vi "sCombine Slow.vi"(1 "HV Cluster":T2={"HV Power On/Off"=[], "Set Voltage"=[], "HV Tolerance (%)"=1.0}, 2 "Rad7 On?":bool, 3 "Slow Cluster":T1) -> (0 "Slow Cluster 2":T1)   [LabVIEW 2012]
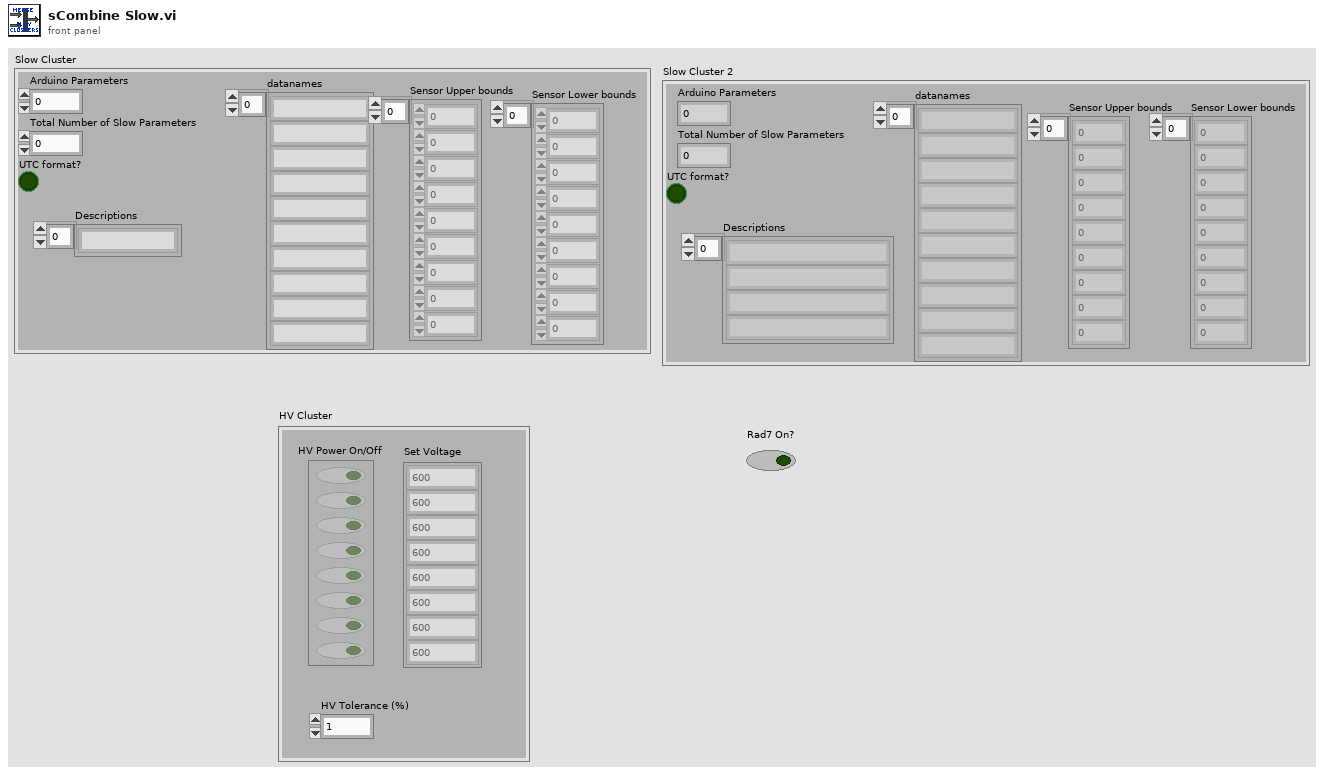
[diagram p1: front panel]
types:
  T1 = cluster{"Arduino Parameters":dbl, "Total Number of Slow Parameters":i32, "UTC format?":bool, "Sensor Upper bounds":i32[], "Sensor Lower bounds":i32[], "Descriptions":string[], "datanames":string[]}
  T2 = cluster{"HV Power On/Off":bool[], "Set Voltage":string[], "HV Tolerance (%)":dbl}
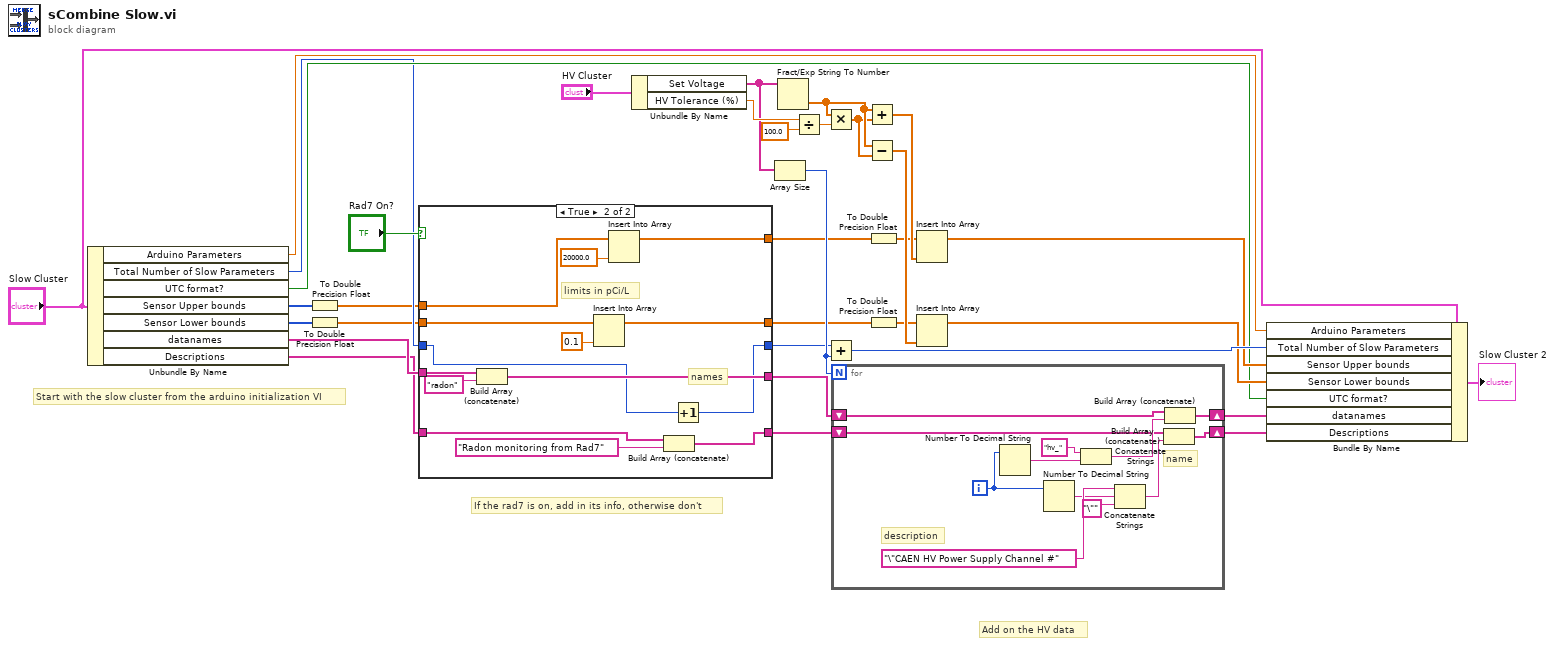
[diagram p0: block diagram]
diagram:
  # "Add on the HV data"
  # "If the rad7 is on, add in its info, otherwise don't"
  # "Start with the slow cluster from the arduino initialization VI"
  n1 = Unbundle By Name("Slow Cluster") -> ("Arduino Parameters"=w16:dbl, "Total Number of Slow Parameters"=w8:i32, "UTC format?"=w20:bool, "Sensor Upper bounds"=w4:i32[], "Sensor Lower bounds"=w3:i32[], "datanames"=w12:string[], "Descriptions"=w10:string[])
  n2 = To Double Precision Float(number=w4) -> (double precision float=w2:dbl[])
  n3 = To Double Precision Float(number=w3) -> (double precision float=w1:dbl[])
  n4 = case shown="True" "Rad7 On?" {
    tunnel: w12 -> [w39 w53]
    tunnel: [w39 w51] -> w11
    tunnel: w10 -> [w38 w49]
    tunnel: [w38 w48] -> w9
    tunnel: w8 -> [w37 w47]
    tunnel: [w37 w46] -> w7
    tunnel: w2 -> [w36 w45]
    tunnel: w1 -> [w35 w44]
    tunnel: [w36 w43] -> w6
    tunnel: [w35 w42] -> w5
    frame False {
    }
    frame True {
      # "limits in pCi/L"
      # "names"
      n5 = Build Array (concatenate)(w53, "radon" ("string")) -> (w51:string[])
      n6 = Insert Into Array(array=w44, new element=0.1 ("new element/subarray")) -> (w42:dbl[])  [unwired: 1 in]
      n7 = Insert Into Array(array=w45, new element=20000.0 ("new element/subarray")) -> (w43:dbl[])  [unwired: 1 in]
      n8 = Build Array (concatenate)(w49, "Radon monitoring from Rad7" ("string")) -> (w48:string[])
      n9 = Increment(x=w47) -> (x+1=w46:i32)
    }
  }
  n10 = Unbundle By Name("HV Cluster") -> ("Set Voltage"=w24:string[], "HV Tolerance (%)"=w30:dbl)
  n11 = Array Size(array=w24) -> (size(s)=w17:i32)
  n12 = Fract/Exp String To Number(string=w24) -> (number=w34:dbl[])  [unwired: 3 in, 1 out]
  n13 = Divide(x=w30, y=100.0) -> (x/y=w28:dbl)
  n14 = Multiply(x=w34, y=w28) -> (x*y=w33:dbl[])
  n15 = Add(x=w7, y=w17) -> (x+y=w23:i32)
  n16 = for {
    N: w17 -> [_]
    shift-right: [w59] -> w19
    shift-left: w11 -> [w61]
    shift-right: [w56] -> w18
    shift-left: w9 -> [w58]
    i -> [w55]
    # "description"
    # "name"
    n17 = Number To Decimal String(number=w55) -> (decimal integer string=w64:string)  [unwired: 1 in]
    n18 = Number To Decimal String(number=w55) -> (decimal integer string=w62:string)  [unwired: 1 in]
    n19 = Concatenate Strings("hv_", w64) -> (w60:string)
    n20 = Concatenate Strings("\"CAEN HV Power Supply Channel #", w62, "\"" ("element")) -> (w57:string)
    n21 = Build Array (concatenate)(w58, w57) -> (w56:string[])
    n22 = Build Array (concatenate)(w61, w60) -> (w59:string[])
  }
  n23 = Add(x=w34, y=w33) -> (x+y=w32:dbl[])
  n24 = Subtract(x=w34, y=w33) -> (x-y=w31:dbl[])
  n25 = To Double Precision Float(number=w6) -> (double precision float=w27:dbl[])
  n26 = To Double Precision Float(number=w5) -> (double precision float=w26:dbl[])
  n27 = Insert Into Array(array=w27, new element=w32) -> (w22:dbl[])  [unwired: 1 in]
  n28 = Insert Into Array(array=w26, new element=w31) -> (w21:dbl[])  [unwired: 1 in]
  n29 = Bundle By Name(cluster="Slow Cluster", "Arduino Parameters"=w16, "Total Number of Slow Parameters"=w23, "Sensor Upper bounds"=w22, "Sensor Lower bounds"=w21, "UTC format?"=w20, "datanames"=w19, "Descriptions"=w18) -> (→"Slow Cluster 2":T1)
